vi "Write Status Error Channel Data References.vi"(8 "error in (no error)":errorcluster, 10 "status error channel data references":T2 {"specific errors"."timeout" format="%.0x"; "specific errors"."bit timing" format="%.0x"; "specific errors"."long word" format="%.0x"; "specific errors"."parity" format="%.0x"; "specific errors"."gap" format="%.0x"; "receiving" format="%.0x"}, 11 "Ballard ARINC-429 Rx Execution Unit in":refnum<class "Ballard ARINC-429 Rx Execution Unit.lvclass">) -> (0 "error out":errorcluster, 3 "Ballard ARINC-429 Rx Execution Unit out":refnum<class "Ballard ARINC-429 Rx Execution Unit.lvclass">)   [LabVIEW 2020, in "Ballard ARINC 429 Engine.lvlib" / "Implementation.lvlib" / "Ballard ARINC-429 Rx Execution Unit.lvclass"]
uses:
  Ballard ARINC-429 Rx Execution Unit.lvclass
  <vilib>/NI VeriStand/Custom Device API/Data Reference.ctl
  Ballard ARINC-429 Rx Execution Unit.lvclass/Ballard ARINC-429 Rx Execution Unit.ctl
  <vilib>/NI VeriStand/Custom Device API/Custom Device API.lvlib
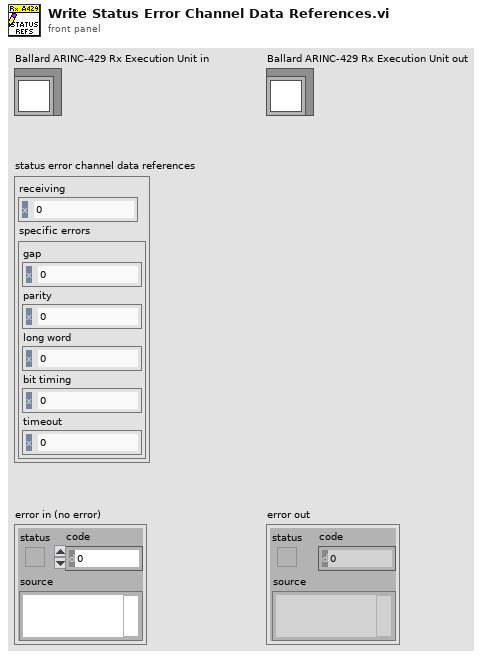
[diagram p1: front panel]
types:
  T1 = typedef "Custom Device API.lvlib/Data Reference.ctl" = i32
  T2 = cluster{"receiving":T1, "specific errors":cluster{"gap":T1, "parity":T1, "long word ":T1, "bit timing":T1, "timeout":T1}}
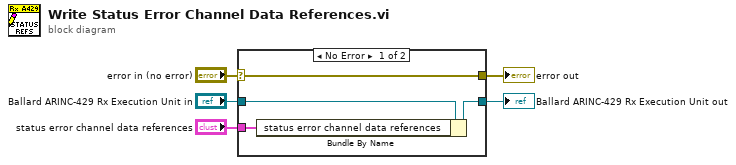
[diagram p0: block diagram]
diagram:
  n1 = case shown="No Error" "error in (no error)" {
    selector: "error in (no error)" -> [w9 w10]
    tunnel: [w9 w10] -> w4
    tunnel: [w6 w11] -> w2
    tunnel: "Ballard ARINC-429 Rx Execution Unit in" -> [w8 w11]
    tunnel: "status error channel data references" -> [w7 _]
    frame No Error {
      n2 = Bundle By Name(cluster=w8, "status error channel data references"=w7) -> (w6:refnum<class "Ballard ARINC-429 Rx Execution Unit.lvclass">)
    }
    frame Error {
    }
  }
  "error out" <- w4
  "Ballard ARINC-429 Rx Execution Unit out" <- w2
